vi "ZK流程读取.vi"(7 "是否启用通讯通知":bool, 8 "error in (no error)":errorcluster, 11 "Slave ID":T2) -> (0 "error out":errorcluster, 3 "流程":T1 {"进样流程"."进样流程-进样"."步骤二："."功能" items=["加标", "进样", "排液", "搅拌", "定量", "延时"]; "进样流程"."进样流程-进样"."步骤一："."功能" items=["加标", "进样", "排液", "搅拌", "定量", "延时"]; "进样流程"."进样流程-进样"."步骤四："."功能" items=["加标", "进样", "排液", "搅拌", "定量", "延时"]; "进样流程"."进样流程-进样"."步骤三："."功能" items=["加标", "进样", "排液", "搅拌", "定量", "延时"]; "进样流程"."进样流程-进样"."步骤六："."功能" items=["加标", "进样", "排液", "搅拌", "定量", "延时"]; "进样流程"."进样流程-进样"."步骤五："."功能" items=["加标", "进样", "排液", "搅拌", "定量", "延时"]; "进样流程"."进样流程-进样"."步骤八："."功能" items=["加标", "进样", "排液", "搅拌", "定量", "延时"]; "进样流程"."进样流程-进样"."步骤七："."功能" items=["加标", "进样", "排液", "搅拌", "定量", "延时"]; "进样流程"."进样流程-进样"."步骤十："."功能" items=["加标", "进样", "排液", "搅拌", "定量", "延时"]; "进样流程"."进样流程-进样"."步骤九："."功能" items=["加标", "进样", "排液", "搅拌", "定量", "延时"]; "进样流程"."进样流程-润洗"."步骤二："."功能" items=["加标", "进样", "排液", "搅拌", "定量", "延时"]; "进样流程"."进样流程-润洗"."步骤一："."功能" items=["加标", "进样", "排液", "搅拌", "定量", "延时"]; "进样流程"."进样流程-润洗"."步骤四："."功能" items=["加标", "进样", "排液", "搅拌", "定量", "延时"]; "进样流程"."进样流程-润洗"."步骤三："."功能" items=["加标", "进样", "排液", "搅拌", "定量", "延时"]; "进样流程"."进样流程-润洗"."步骤六："."功能" items=["加标", "进样", "排液", "搅拌", "定量", "延时"]; "进样流程"."进样流程-润洗"."步骤五："."功能" items=["加标", "进样", "排液", "搅拌", "定量", "延时"]; "进样流程"."进样流程-润洗"."步骤八："."功能" items=["加标", "进样", "排液", "搅拌", "定量", "延时"]; "进样流程"."进样流程-润洗"."步骤七："."功能" items=["加标", "进样", "排液", "搅拌", "定量", "延时"]; "进样流程"."进样流程-润洗"."步骤十："."功能" items=["加标", "进样", "排液", "搅拌", "定量", "延时"]; "进样流程"."进样流程-润洗"."步骤九："."功能" items=["加标", "进样", "排液", "搅拌", "定量", "延时"]; "排液流程"."步骤二："."功能" items=["加标", "进样", "排液", "搅拌", "定量", "延时"]; "排液流程"."步骤一："."功能" items=["加标", "进样", "排液", "搅拌", "定量", "延时"]; "排液流程"."步骤四："."功能" items=["加标", "进样", "排液", "搅拌", "定量", "延时"]; "排液流程"."步骤三："."功能" items=["加标", "进样", "排液", "搅拌", "定量", "延时"]; "排液流程"."步骤六："."功能" items=["加标", "进样", "排液", "搅拌", "定量", "延时"]; "排液流程"."步骤五："."功能" items=["加标", "进样", "排液", "搅拌", "定量", "延时"]; "排液流程"."步骤八："."功能" items=["加标", "进样", "排液", "搅拌", "定量", "延时"]; "排液流程"."步骤七："."功能" items=["加标", "进样", "排液", "搅拌", "定量", "延时"]; "排液流程"."步骤十："."功能" items=["加标", "进样", "排液", "搅拌", "定量", "延时"]; "排液流程"."步骤九："."功能" items=["加标", "进样", "排液", "搅拌", "定量", "延时"]; "加标流程"."加标流程-加标"."步骤二："."功能" items=["加标", "进样", "排液", "搅拌", "定量", "延时"]; "加标流程"."加标流程-加标"."步骤一："."功能" items=["加标", "进样", "排液", "搅拌", "定量", "延时"]; "加标流程"."加标流程-加标"."步骤四："."功能" items=["加标", "进样", "排液", "搅拌", "定量", "延时"]; "加标流程"."加标流程-加标"."步骤三："."功能" items=["加标", "进样", "排液", "搅拌", "定量", "延时"]; "加标流程"."加标流程-加标"."步骤六："."功能" items=["加标", "进样", "排液", "搅拌", "定量", "延时"]; "加标流程"."加标流程-加标"."步骤五："."功能" items=["加标", "进样", "排液", "搅拌", "定量", "延时"]; "加标流程"."加标流程-加标"."步骤八："."功能" items=["加标", "进样", "排液", "搅拌", "定量", "延时"]; "加标流程"."加标流程-加标"."步骤七："."功能" items=["加标", "进样", "排液", "搅拌", "定量", "延时"]; "加标流程"."加标流程-加标"."步骤十："."功能" items=["加标", "进样", "排液", "搅拌", "定量", "延时"]; "加标流程"."加标流程-加标"."步骤九："."功能" items=["加标", "进样", "排液", "搅拌", "定量", "延时"]; "加标流程"."加标流程-定量"."步骤二："."功能" items=["加标", "进样", "排液", "搅拌", "定量", "延时"]; "加标流程"."加标流程-定量"."步骤一："."功能" items=["加标", "进样", "排液", "搅拌", "定量", "延时"]; "加标流程"."加标流程-定量"."步骤四："."功能" items=["加标", "进样", "排液", "搅拌", "定量", "延时"]; "加标流程"."加标流程-定量"."步骤三："."功能" items=["加标", "进样", "排液", "搅拌", "定量", "延时"]; "加标流程"."加标流程-定量"."步骤六："."功能" items=["加标", "进样", "排液", "搅拌", "定量", "延时"]; "加标流程"."加标流程-定量"."步骤五："."功能" items=["加标", "进样", "排液", "搅拌", "定量", "延时"]; "加标流程"."加标流程-定量"."步骤八："."功能" items=["加标", "进样", "排液", "搅拌", "定量", "延时"]; "加标流程"."加标流程-定量"."步骤七："."功能" items=["加标", "进样", "排液", "搅拌", "定量", "延时"]; "加标流程"."加标流程-定量"."步骤十："."功能" items=["加标", "进样", "排液", "搅拌", "定量", "延时"]; "加标流程"."加标流程-定量"."步骤九："."功能" items=["加标", "进样", "排液", "搅拌", "定量", "延时"]; "加标流程"."加标流程-进样"."步骤二："."功能" items=["加标", "进样", "排液", "搅拌", "定量", "延时"]; "加标流程"."加标流程-进样"."步骤一："."功能" items=["加标", "进样", "排液", "搅拌", "定量", "延时"]; "加标流程"."加标流程-进样"."步骤四："."功能" items=["加标", "进样", "排液", "搅拌", "定量", "延时"]; "加标流程"."加标流程-进样"."步骤三："."功能" items=["加标", "进样", "排液", "搅拌", "定量", "延时"]; "加标流程"."加标流程-进样"."步骤六："."功能" items=["加标", "进样", "排液", "搅拌", "定量", "延时"]; "加标流程"."加标流程-进样"."步骤五："."功能" items=["加标", "进样", "排液", "搅拌", "定量", "延时"]; "加标流程"."加标流程-进样"."步骤八："."功能" items=["加标", "进样", "排液", "搅拌", "定量", "延时"]; "加标流程"."加标流程-进样"."步骤七："."功能" items=["加标", "进样", "排液", "搅拌", "定量", "延时"]; "加标流程"."加标流程-进样"."步骤十："."功能" items=["加标", "进样", "排液", "搅拌", "定量", "延时"]; "加标流程"."加标流程-进样"."步骤九："."功能" items=["加标", "进样", "排液", "搅拌", "定量", "延时"]; "加标流程"."加标流程-润洗"."步骤二："."功能" items=["加标", "进样", "排液", "搅拌", "定量", "延时"]; "加标流程"."加标流程-润洗"."步骤一："."功能" items=["加标", "进样", "排液", "搅拌", "定量", "延时"]; "加标流程"."加标流程-润洗"."步骤四："."功能" items=["加标", "进样", "排液", "搅拌", "定量", "延时"]; "加标流程"."加标流程-润洗"."步骤三："."功能" items=["加标", "进样", "排液", "搅拌", "定量", "延时"]; "加标流程"."加标流程-润洗"."步骤六："."功能" items=["加标", "进样", "排液", "搅拌", "定量", "延时"]; "加标流程"."加标流程-润洗"."步骤五："."功能" items=["加标", "进样", "排液", "搅拌", "定量", "延时"]; "加标流程"."加标流程-润洗"."步骤八："."功能" items=["加标", "进样", "排液", "搅拌", "定量", "延时"]; "加标流程"."加标流程-润洗"."步骤七："."功能" items=["加标", "进样", "排液", "搅拌", "定量", "延时"]; "加标流程"."加标流程-润洗"."步骤十："."功能" items=["加标", "进样", "排液", "搅拌", "定量", "延时"]; "加标流程"."加标流程-润洗"."步骤九："."功能" items=["加标", "进样", "排液", "搅拌", "定量", "延时"]; "加标润洗流程"."步骤二："."功能" items=["加标", "进样", "排液", "搅拌", "定量", "延时"]; "加标润洗流程"."步骤一："."功能" items=["加标", "进样", "排液", "搅拌", "定量", "延时"]; "加标润洗流程"."步骤四："."功能" items=["加标", "进样", "排液", "搅拌", "定量", "延时"]; "加标润洗流程"."步骤三："."功能" items=["加标", "进样", "排液", "搅拌", "定量", "延时"]; "加标润洗流程"."步骤六："."功能" items=["加标", "进样", "排液", "搅拌", "定量", "延时"]; "加标润洗流程"."步骤五："."功能" items=["加标", "进样", "排液", "搅拌", "定量", "延时"]; "加标润洗流程"."步骤八："."功能" items=["加标", "进样", "排液", "搅拌", "定量", "延时"]; "加标润洗流程"."步骤七："."功能" items=["加标", "进样", "排液", "搅拌", "定量", "延时"]; "加标润洗流程"."步骤十："."功能" items=["加标", "进样", "排液", "搅拌", "定量", "延时"]; "加标润洗流程"."步骤九："."功能" items=["加标", "进样", "排液", "搅拌", "定量", "延时"]; "水样润洗流程"."步骤二："."功能" items=["加标", "进样", "排液", "搅拌", "定量", "延时"]; "水样润洗流程"."步骤一："."功能" items=["加标", "进样", "排液", "搅拌", "定量", "延时"]; "水样润洗流程"."步骤四："."功能" items=["加标", "进样", "排液", "搅拌", "定量", "延时"]; "水样润洗流程"."步骤三："."功能" items=["加标", "进样", "排液", "搅拌", "定量", "延时"]; "水样润洗流程"."步骤六："."功能" items=["加标", "进样", "排液", "搅拌", "定量", "延时"]; "水样润洗流程"."步骤五："."功能" items=["加标", "进样", "排液", "搅拌", "定量", "延时"]; "水样润洗流程"."步骤八："."功能" items=["加标", "进样", "排液", "搅拌", "定量", "延时"]; "水样润洗流程"."步骤七："."功能" items=["加标", "进样", "排液", "搅拌", "定量", "延时"]; "水样润洗流程"."步骤十："."功能" items=["加标", "进样", "排液", "搅拌", "定量", "延时"]; "水样润洗流程"."步骤九："."功能" items=["加标", "进样", "排液", "搅拌", "定量", "延时"]})   [LabVIEW 2016, in "质控单元V4.lvlib"]
uses:
  <vilib>/Plasmionique/MB Master/MB_Master/MB_Master.lvclass
  <vilib>/Plasmionique/MB Master/MB Master.lvlib
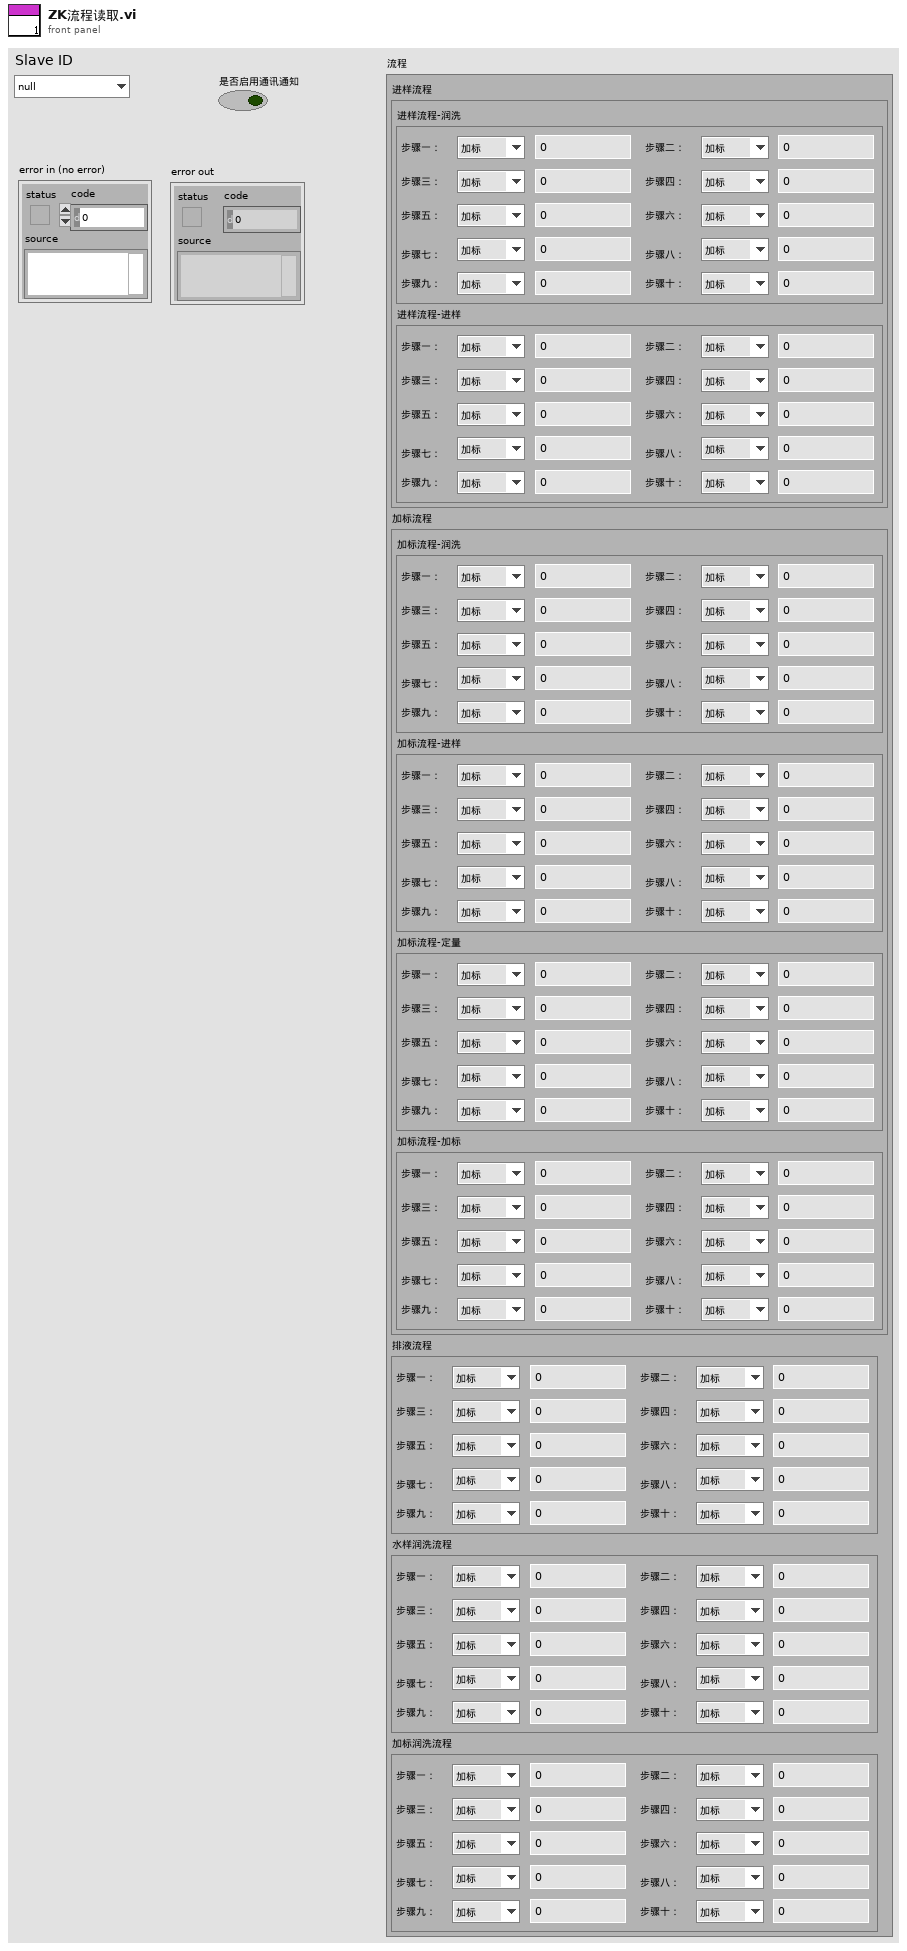
[diagram p1: front panel]
types:
  T1 = cluster{"进样流程":cluster{"进样流程-润洗":cluster{"步骤一：":cluster{"功能":u16, "值":sgl}, "步骤二：":cluster{"功能":u16, "值":sgl}, "步骤三：":cluster{"功能":u16, "值":sgl}, "步骤四：":cluster{"功能":u16, "值":sgl}, "步骤五：":cluster{"功能":u16, "值":sgl}, "步骤六：":cluster{"功能":u16, "值":sgl}, "步骤七：":cluster{"功能":u16, "值":sgl}, "步骤八：":cluster{"功能":u16, "值":sgl}, "步骤九：":cluster{"功能":u16, "值":sgl}, "步骤十：":cluster{"功能":u16, "值":sgl}}, "进样流程-进样":cluster{"步骤一：":cluster{"功能":u16, "值":sgl}, "步骤二：":cluster{"功能":u16, "值":sgl}, "步骤三：":cluster{"功能":u16, "值":sgl}, "步骤四：":cluster{"功能":u16, "值":sgl}, "步骤五：":cluster{"功能":u16, "值":sgl}, "步骤六：":cluster{"功能":u16, "值":sgl}, "步骤七：":cluster{"功能":u16, "值":sgl}, "步骤八：":cluster{"功能":u16, "值":sgl}, "步骤九：":cluster{"功能":u16, "值":sgl}, "步骤十：":cluster{"功能":u16, "值":sgl}}}, "加标流程":cluster{"加标流程-润洗":cluster{"步骤一：":cluster{"功能":u16, "值":sgl}, "步骤二：":cluster{"功能":u16, "值":sgl}, "步骤三：":cluster{"功能":u16, "值":sgl}, "步骤四：":cluster{"功能":u16, "值":sgl}, "步骤五：":cluster{"功能":u16, "值":sgl}, "步骤六：":cluster{"功能":u16, "值":sgl}, "步骤七：":cluster{"功能":u16, "值":sgl}, "步骤八：":cluster{"功能":u16, "值":sgl}, "步骤九：":cluster{"功能":u16, "值":sgl}, "步骤十：":cluster{"功能":u16, "值":sgl}}, "加标流程-进样":cluster{"步骤一：":cluster{"功能":u16, "值":sgl}, "步骤二：":cluster{"功能":u16, "值":sgl}, "步骤三：":cluster{"功能":u16, "值":sgl}, "步骤四：":cluster{"功能":u16, "值":sgl}, "步骤五：":cluster{"功能":u16, "值":sgl}, "步骤六：":cluster{"功能":u16, "值":sgl}, "步骤七：":cluster{"功能":u16, "值":sgl}, "步骤八：":cluster{"功能":u16, "值":sgl}, "步骤九：":cluster{"功能":u16, "值":sgl}, "步骤十：":cluster{"功能":u16, "值":sgl}}, "加标流程-定量":cluster{"步骤一：":cluster{"功能":u16, "值":sgl}, "步骤二：":cluster{"功能":u16, "值":sgl}, "步骤三：":cluster{"功能":u16, "值":sgl}, "步骤四：":cluster{"功能":u16, "值":sgl}, "步骤五：":cluster{"功能":u16, "值":sgl}, "步骤六：":cluster{"功能":u16, "值":sgl}, "步骤七：":cluster{"功能":u16, "值":sgl}, "步骤八：":cluster{"功能":u16, "值":sgl}, "步骤九：":cluster{"功能":u16, "值":sgl}, "步骤十：":cluster{"功能":u16, "值":sgl}}, "加标流程-加标":cluster{"步骤一：":cluster{"功能":u16, "值":sgl}, "步骤二：":cluster{"功能":u16, "值":sgl}, "步骤三：":cluster{"功能":u16, "值":sgl}, "步骤四：":cluster{"功能":u16, "值":sgl}, "步骤五：":cluster{"功能":u16, "值":sgl}, "步骤六：":cluster{"功能":u16, "值":sgl}, "步骤七：":cluster{"功能":u16, "值":sgl}, "步骤八：":cluster{"功能":u16, "值":sgl}, "步骤九：":cluster{"功能":u16, "值":sgl}, "步骤十：":cluster{"功能":u16, "值":sgl}}}, "排液流程":cluster{"步骤一：":cluster{"功能":u16, "值":sgl}, "步骤二：":cluster{"功能":u16, "值":sgl}, "步骤三：":cluster{"功能":u16, "值":sgl}, "步骤四：":cluster{"功能":u16, "值":sgl}, "步骤五：":cluster{"功能":u16, "值":sgl}, "步骤六：":cluster{"功能":u16, "值":sgl}, "步骤七：":cluster{"功能":u16, "值":sgl}, "步骤八：":cluster{"功能":u16, "值":sgl}, "步骤九：":cluster{"功能":u16, "值":sgl}, "步骤十：":cluster{"功能":u16, "值":sgl}}, "水样润洗流程":cluster{"步骤一：":cluster{"功能":u16, "值":sgl}, "步骤二：":cluster{"功能":u16, "值":sgl}, "步骤三：":cluster{"功能":u16, "值":sgl}, "步骤四：":cluster{"功能":u16, "值":sgl}, "步骤五：":cluster{"功能":u16, "值":sgl}, "步骤六：":cluster{"功能":u16, "值":sgl}, "步骤七：":cluster{"功能":u16, "值":sgl}, "步骤八：":cluster{"功能":u16, "值":sgl}, "步骤九：":cluster{"功能":u16, "值":sgl}, "步骤十：":cluster{"功能":u16, "值":sgl}}, "加标润洗流程":cluster{"步骤一：":cluster{"功能":u16, "值":sgl}, "步骤二：":cluster{"功能":u16, "值":sgl}, "步骤三：":cluster{"功能":u16, "值":sgl}, "步骤四：":cluster{"功能":u16, "值":sgl}, "步骤五：":cluster{"功能":u16, "值":sgl}, "步骤六：":cluster{"功能":u16, "值":sgl}, "步骤七：":cluster{"功能":u16, "值":sgl}, "步骤八：":cluster{"功能":u16, "值":sgl}, "步骤九：":cluster{"功能":u16, "值":sgl}, "步骤十：":cluster{"功能":u16, "值":sgl}}}
  T2 = typedef "质控单元V4.lvlib/质控slave id.ctl" = enum16{"null", "氨氮", "总磷", "总氮", "CODMn", "CODCr"}
  T3 = cluster{"[0]":cluster{"功能":u16, "值":sgl}, "[1]":cluster{"功能":u16, "值":sgl}, "[2]":cluster{"功能":u16, "值":sgl}, "[3]":cluster{"功能":u16, "值":sgl}, "[4]":cluster{"功能":u16, "值":sgl}, "[5]":cluster{"功能":u16, "值":sgl}, "[6]":cluster{"功能":u16, "值":sgl}, "[7]":cluster{"功能":u16, "值":sgl}, "[8]":cluster{"功能":u16, "值":sgl}, "[9]":cluster{"功能":u16, "值":sgl}}
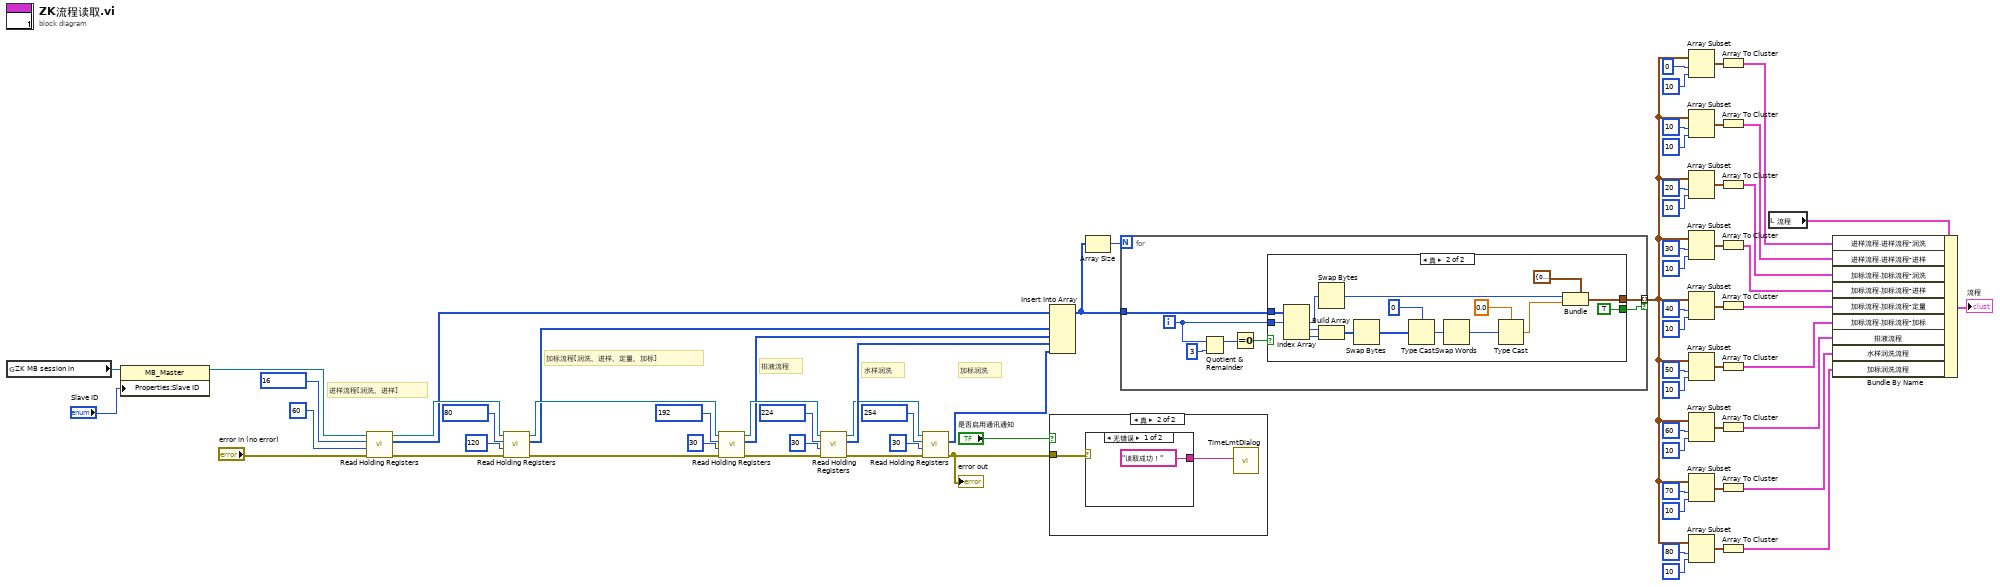
[diagram p0: block diagram]
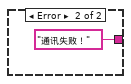
[diagram p4: hidden frame]
diagram:
  # "加标润洗"
  # "水样润洗"
  # "排液流程"
  # "加标流程[润洗、进样、定量、加标]"
  # "进样流程[润洗、进样]"
  n1 = global read "ZK非断电保存全局变量.vi" "ZK MB session in"() -> (w1:refnum<class "MB_Master.lvclass">)
  n2 = property class="MB_Master"(reference=w1, "Properties:Slave ID"="Slave ID") -> (reference out=w68:refnum<class "MB_Master.lvclass">)  [unwired: 1 in, 1 out]
  n3 = call <vilib>:"Read Holding Registers.vi"("error in (no error)"="error in (no error)", "quantity"=u16 60, "starting address"=u16 16, "MB session in"=w68) -> ("error out"=w32:errorcluster, "Registers"=w26:u16[], "MB session out"=w29:refnum<class "MB_Master.lvclass">)  [unwired: 5 in]
  n4 = call <vilib>:"Read Holding Registers.vi"("error in (no error)"=w32, "quantity"=u16 120, "starting address"=u16 80, "MB session in"=w29) -> ("error out"=w31:errorcluster, "Registers"=w24:u16[], "MB session out"=w28:refnum<class "MB_Master.lvclass">)  [unwired: 5 in]
  n5 = call <vilib>:"Read Holding Registers.vi"("error in (no error)"=w31, "quantity"=u16 30, "starting address"=u16 192, "MB session in"=w28) -> ("error out"=w30:errorcluster, "Registers"=w23:u16[], "MB session out"=w27:refnum<class "MB_Master.lvclass">)  [unwired: 5 in]
  n6 = call <vilib>:"Read Holding Registers.vi"("error in (no error)"=w30, "quantity"=u16 30, "starting address"=u16 224, "MB session in"=w27) -> ("error out"=w11:errorcluster, "Registers"=w22:u16[], "MB session out"=w10:refnum<class "MB_Master.lvclass">)  [unwired: 5 in]
  n7 = call <vilib>:"Read Holding Registers.vi"("error in (no error)"=w11, "quantity"=u16 30, "starting address"=u16 254, "MB session in"=w10) -> ("error out"=w6:errorcluster, "Registers"=w7:u16[])  [unwired: 5 in, 1 out]
  "error out" <- w6
  n8 = Insert Into Array(array=w26, new element #1=w24, new element #2=w23, new element #3=w22, new element #4=w7) -> (w25:u16[])  [unwired: 1 in]
  n9 = case shown="真" "是否启用通讯通知" {
    tunnel: w6 -> [_ w72]
    frame False {
    }
    frame True {
      n10 = case shown="无错误" w72 {
        tunnel: ["读取成功！" "通讯失败！"] -> w71
        frame No Error {
        }
        frame Error {
        }
      }
      n11 = call "TimeLmtDialog.vi"("Infoin"=w71) -> ()  [unwired: 11 in]
    }
  }
  n12 = Array Size(array=w25) -> (size(s)=w64:i32)
  n13 = for {
    N: w64 -> [_]
    tunnel: w25 -> [w80]
    tunnel: [w79] -> w5 mode=indexing if=w76
    i -> [w75]
    n14 = Quotient & Remainder(x=w75, y=3) -> (x-y*floor(x/y)=w78:i32)  [unwired: 1 out]
    n15 = Equal To 0?(x=w78) -> (x = 0?=w77:bool)
    n16 = case shown="真" w77 {
      tunnel: w80 -> [_ w97]
      tunnel: w75 -> [_ w96]
      tunnel: [_ w83] -> w79
      tunnel: [_ TRUE] -> w76
      frame False {
      }
      frame True {
        n17 = Index Array(array=w97, index #1=w96) -> (element #1=w95:u16, element #2=w94:u16, element #3=w93:u16)  [unwired: 2 in]
        n18 = Swap Bytes(anything=w95) -> (byte swapped=w85:u16)
        n19 = Build Array(w94, w93) -> (w87:u16[])
        n20 = Swap Bytes(anything=w87) -> (byte swapped=w90:u16[])
        n21 = Type Cast(type=u32 0, x=w90) -> (*(type *) &x=w88:u32)
        n22 = Swap Words(1:w88) -> (0:w89:u32)
        n23 = Type Cast(type=sgl 0.0, x=w89) -> (*(type *) &x=w86:sgl)
        n24 = Bundle(cluster=cluster{"功能":u16, "值":sgl} {"功能"=0, "值"=0.0} ("簇"), "功能"=w85, "值"=w86) -> (w83:cluster{"功能":u16, "值":sgl})
      }
    }
  }
  n25 = Array Subset(array=w5, index=0 ("索引"), length=10 ("长度")) -> (w57:cluster{"功能":u16, "值":sgl}[])
  n26 = Array Subset(array=w5, index=10 ("索引"), length=10 ("长度")) -> (w13:cluster{"功能":u16, "值":sgl}[])
  n27 = Array Subset(array=w5, index=20 ("索引"), length=10 ("长度")) -> (w55:cluster{"功能":u16, "值":sgl}[])
  n28 = Array Subset(array=w5, index=30 ("索引"), length=10 ("长度")) -> (w50:cluster{"功能":u16, "值":sgl}[])
  n29 = Array Subset(array=w5, index=40 ("索引"), length=10 ("长度")) -> (w49:cluster{"功能":u16, "值":sgl}[])
  n30 = Array Subset(array=w5, index=50 ("索引"), length=10 ("长度")) -> (w44:cluster{"功能":u16, "值":sgl}[])
  n31 = Array Subset(array=w5, index=60 ("索引"), length=10 ("长度")) -> (w34:cluster{"功能":u16, "值":sgl}[])
  n32 = Array Subset(array=w5, index=70 ("索引"), length=10 ("长度")) -> (w60:cluster{"功能":u16, "值":sgl}[])
  n33 = Array Subset(array=w5, index=80 ("索引"), length=10 ("长度")) -> (w39:cluster{"功能":u16, "值":sgl}[])
  n34 = Array To Cluster(array=w57) -> (cluster=w56:T3)
  n35 = Array To Cluster(array=w13) -> (cluster=w12:T3)
  n36 = Array To Cluster(array=w55) -> (cluster=w43:T3)
  n37 = Array To Cluster(array=w50) -> (cluster=w42:T3)
  n38 = Array To Cluster(array=w49) -> (cluster=w41:T3)
  n39 = Array To Cluster(array=w44) -> (cluster=w40:T3)
  n40 = Array To Cluster(array=w34) -> (cluster=w33:T3)
  n41 = Array To Cluster(array=w60) -> (cluster=w3:T3)
  n42 = Array To Cluster(array=w39) -> (cluster=w2:T3)
  n43 = local read "流程"() -> (w63:T1)
  n44 = Bundle By Name(cluster=w63, "进样流程.进样流程-润洗"=w56, "进样流程.进样流程-进样"=w12, "加标流程.加标流程-润洗"=w43, "加标流程.加标流程-进样"=w42, "加标流程.加标流程-定量"=w41, "加标流程.加标流程-加标"=w40, "排液流程"=w33, "水样润洗流程"=w3, "加标润洗流程"=w2) -> (→"流程":T1)
